vi "Prompt Break Out.vi"(8 "error in (no error)":errorcluster) -> (0 "error out":errorcluster)   [LabVIEW 2018, in "Controller (Host).lvlib"]
doc: "This subVI enqueues the named action in to the communications queue along with the input data."
uses:
  Controller (Host).lvlib
  Private Controls/Module Action.ctl
  Private Controls/Module Data.ctl
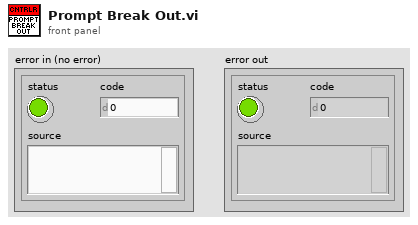
[diagram p1: front panel]
types:
  T1 = typedef "Controller (Host).lvlib/Module Data.ctl" = cluster{"Data":variant, "Action":T2}
  T2 = typedef "Controller (Host).lvlib/Module Action.ctl" = enum8{"Timeout", "Init", "Error", "Exit", "Set cRIO Connected Status", "Prompt Login", "Prompt Main Menu", "Prompt APU Select", "Prompt Operation Select", "Prompt SubTests Select", "Prompt Break Out", "Calibration", "Testing", "Load User Info", "Set Instr Init Status", "Load APU Setup Data", "RPM Cross 95Perc Thresh", "Interactive Ctrls Val Change", "Update Report FilePath"}
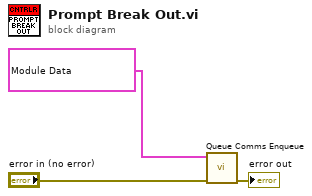
[diagram p0: block diagram]
diagram:
  n1 = call "Queue Comms Enqueue.vi"("error in (no error)"="error in (no error)", "element"=T1 {"Data"=variant, "Action"=enum."Prompt Break Out"}) -> ("error out"=→"error out":errorcluster)  [unwired: 9 in]
